vi "PunkteEntlangVektor.vi"(1 "versatz":cluster{"x":dbl, "y":dbl}={"x"=2.0, "y"=1.0} {"y" format="%.2f"; "x" format="%.2f"}, 2 "vektorstart":cluster{"x":dbl, "y":dbl}={"x"=2.0, "y"=3.0} {"y" format="%.2f"; "x" format="%.2f"}) -> (0 "Array":cluster{"x":i32, "y":i32}[](array[cluster])=[{"x"=2, "y"=3}, {"x"=3, "y"=4}, {"x"=4, "y"=4}])   [LabVIEW 2011]
panel:
  # "Pixelfolge entlang eines vektors, Pixelraster =1 Einheit\nsollte Mindestens 1 element=start zurückliefern!!"
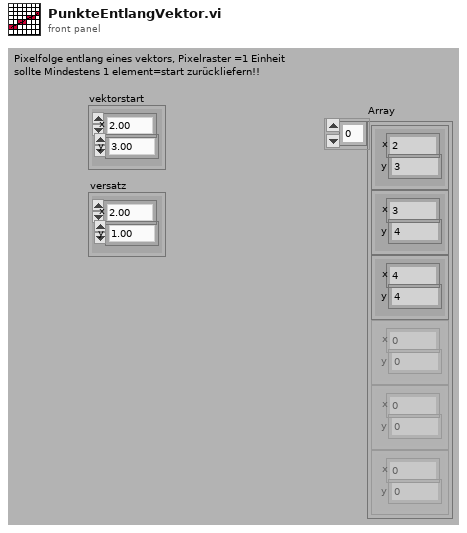
[diagram p1: front panel]
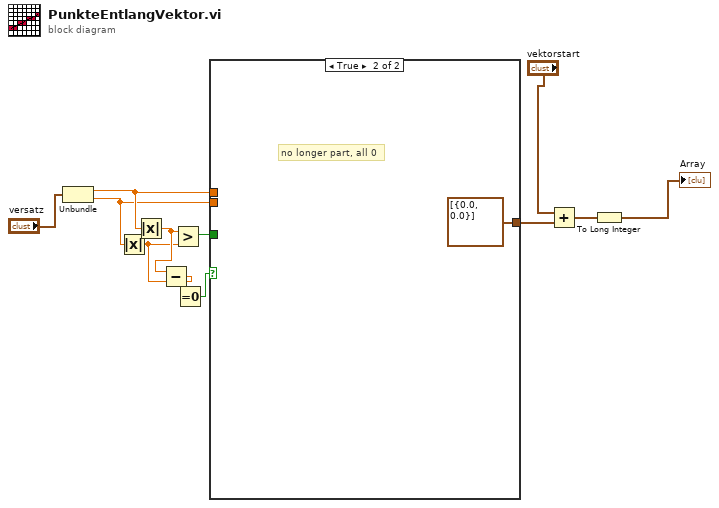
[diagram p0: block diagram]
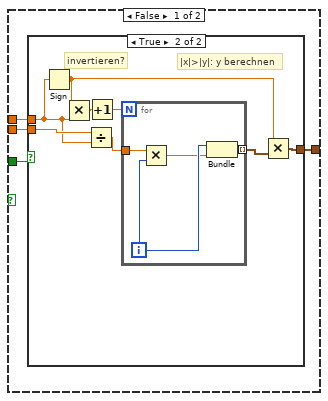
[diagram p2: hidden frame]
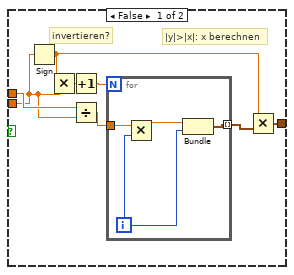
[diagram p3: hidden frame]
diagram:
  n1 = Unbundle("versatz") -> ("x"=w10:dbl, "y"=w9:dbl)
  n2 = Absolute Value(x=w9) -> (abs(x)=w3:dbl)
  n3 = Absolute Value(x=w10) -> (abs(x)=w4:dbl)
  n4 = Subtract(x=w4, y=w3) -> (x-y=w2:dbl)
  n5 = Greater?(x=w4, y=w3) -> (0:w11:bool)
  n6 = Equal To 0?(x=w2) -> (x = 0?=w1:bool)
  n7 = case shown="True" w1 {
    tunnel: w11 -> [w16 _]
    tunnel: w10 -> [w15 _]
    tunnel: w9 -> [w14 _]
    tunnel: [w13 cluster{dbl, dbl}[] [{0.0, 0.0}]] -> w8
    frame False {
      n8 = case shown="True" w16 {
        tunnel: w15 -> [w24 w30]
        tunnel: w14 -> [w17 w36]
        tunnel: [w19 w33] -> w13
        frame False {
          # "invertieren?"
          # "|y|>|x|: x berechnen"
          n9 = Sign(1:w17) -> (0:w21:dbl)
          n10 = Multiply(x=w21, y=w17) -> (x*y=w20:dbl)
          n11 = Increment(x=w20) -> (x+1=w18:dbl)
          n12 = Divide(x=w24, y=w17) -> (x/y=w23:dbl)
          n13 = for {
            N: w18 -> [_]
            tunnel: w23 -> [w28]
            tunnel: [w27] -> w22 mode=indexing
            i -> [w25]
            n14 = Multiply(x=w28, y=w25) -> (x*y=w26:dbl)
            n15 = Bundle(w26, w25) -> (w27:cluster{dbl, i32})  [unwired: 1 out]
          }
          n16 = Multiply(x=w21, y=w22) -> (x*y=w19:cluster{dbl, dbl}[])
        }
        frame True {
          # "invertieren?"
          # "|x|>|y|: y berechnen"
          n17 = Sign(1:w30) -> (0:w32:dbl)
          n18 = Multiply(x=w32, y=w30) -> (x*y=w31:dbl)
          n19 = Divide(x=w36, y=w30) -> (x/y=w35:dbl)
          n20 = Increment(x=w31) -> (x+1=w29:dbl)
          n21 = for {
            N: w29 -> [_]
            tunnel: w35 -> [w40]
            tunnel: [w38] -> w34 mode=indexing
            i -> [w39]
            n22 = Multiply(x=w40, y=w39) -> (x*y=w37:dbl)
            n23 = Bundle(w39, w37) -> (w38:cluster{i32, dbl})  [unwired: 1 out]
          }
          n24 = Multiply(x=w32, y=w34) -> (x*y=w33:cluster{dbl, dbl}[])
        }
      }
    }
    frame True {
      # "no longer part, all 0"
    }
  }
  n25 = Add(x="vektorstart", y=w8) -> (x+y=w6:cluster{dbl, dbl}[])
  n26 = To Long Integer(number=w6) -> (32bit integer=→"Array":cluster{i32, i32}[])
